vi "Convert RawVal to EngineeringUnits.vi"(8 "error in (no error)":errorcluster, 10 "Raw Value In":dbl format="%.3g", 11 "Conversion":T1 {"ScaleOffset" format="%.3f"; "MinEngUnit" format="%.3f"; "MaxEngUnit" format="%.3f"; "MinSignal" format="%.3f"; "MaxSignal" format="%.3f"}) -> (0 "error out":errorcluster, 2 "Engineering Units Out":dbl format="%.3g")   [LabVIEW 2017, in "DAQ.lvclass"]
doc: "Developed by Kevin Thompson\nkevin@thompsonengineering.net\n\nCopyright 2018-2020\nThompson Engineering, LLC"
uses:
  DAQ.lvclass
  DataTypes/TD DataValueConversion--cluster.ctl
  <vilib>/Analysis/NI_AALPro.lvlib
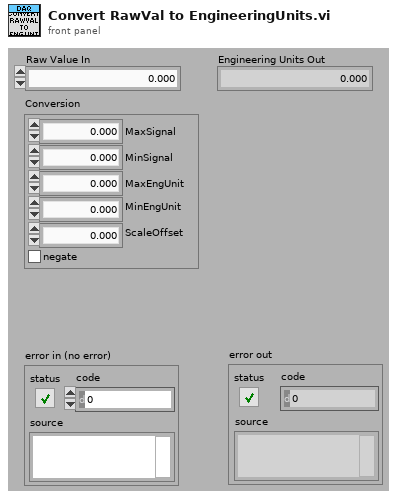
[diagram p1: front panel]
types:
  T1 = typedef "DAQ.lvclass/TD DataValueConversion--cluster.ctl" = cluster{"MaxSignal":dbl, "MinSignal":dbl, "MaxEngUnit":dbl, "MinEngUnit":dbl, "ScaleOffset":dbl, "negate":bool}
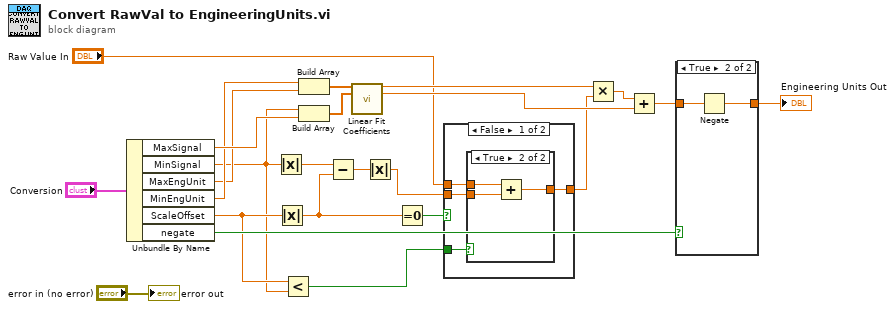
[diagram p0: block diagram]
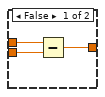
[diagram p2: hidden frame]
diagram:
  n1 = Unbundle By Name("Conversion") -> ("MaxSignal"=w19:dbl, "MinSignal"=w2:dbl, "MaxEngUnit"=w17:dbl, "MinEngUnit"=w18:dbl, "ScaleOffset"=w3:dbl, "negate"=w20:bool)
  n2 = Absolute Value(x=w2) -> (abs(x)=w6:dbl)
  n3 = Absolute Value(x=w3) -> (abs(x)=w5:dbl)
  n4 = Less?(x=w3, y=w2) -> (x < y?=w1:bool)
  n5 = Build Array(w18, w17) -> (w11:dbl[])
  n6 = Build Array(w2, w19) -> (w12:dbl[])
  n7 = Subtract(x=w6, y=w5) -> (x-y=w10:dbl)
  n8 = call <vilib>:"Linear Fit Coefficients.vi"("Y"=w11, "X"=w12) -> ("slope"=w16:dbl, "intercept"=w14:dbl)  [unwired: 11 in, 1 out]
  n9 = Absolute Value(x=w10) -> (abs(x)=w8:dbl)
  n10 = Equal To 0?(x=w5) -> (x = 0?=w4:bool)
  n11 = case shown="False" w4 {
    tunnel: "Raw Value In" -> [w27 w34]
    tunnel: w8 -> [w26 _]
    tunnel: [w25 w34] -> w7
    tunnel: w1 -> [w24 _]
    frame False {
      n12 = case shown="True" w24 {
        tunnel: w27 -> [w30 w33]
        tunnel: w26 -> [w29 w32]
        tunnel: [w28 w31] -> w25
        frame False {
          n13 = Subtract(x=w30, y=w29) -> (x-y=w28:dbl)
        }
        frame True {
          n14 = Add(x=w33, y=w32) -> (x+y=w31:dbl)
        }
      }
    }
    frame True {
    }
  }
  n15 = Multiply(x=w16, y=w7) -> (x*y=w15:dbl)
  n16 = Add(x=w15, y=w14) -> (x+y=w13:dbl)
  n17 = case shown="True" w20 {
    tunnel: [w35 w36] -> w21
    tunnel: w13 -> [w35 w37]
    frame False {
    }
    frame True {
      n18 = Negate(x=w37) -> (-x=w36:dbl)
    }
  }
  "Engineering Units Out" <- w21
  "error out" <- "error in (no error)"
